vi "SetupDefault.vi"(8 "error in (no error)":errorcluster, 10 "Alias":string, 11 "SigGen_NIRF in":refnum<class "SigGen_NIRF.lvclass">) -> (0 "error out":errorcluster, 3 "SigGen_NIRF out":refnum<class "SigGen_NIRF.lvclass">)   [LabVIEW 2014, in "SigGen_NIRF.lvclass"]
uses:
  SigGen_NIRF.lvclass
  SigGen_NIRF.lvclass/SigGen_NIRF.ctl
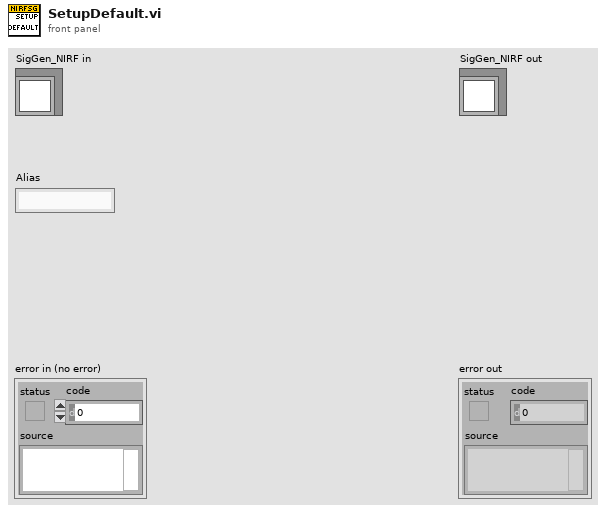
[diagram p1: front panel]
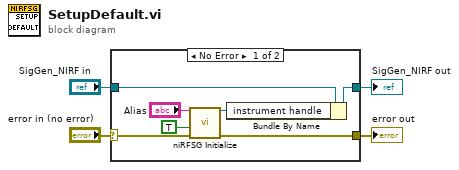
[diagram p0: block diagram]
diagram:
  n1 = case shown="No Error" "error in (no error)" {
    selector: "error in (no error)" -> [w5 w13]
    tunnel: "SigGen_NIRF in" -> [w10 w12]
    tunnel: [w9 w12] -> w3
    tunnel: [w7 w13] -> w2
    frame No Error {
      n2 = call "niRFSG Initialize.vi"("resource name"="Alias", "reset device"=TRUE, "error in"=w5) -> ("instrument handle"=w8:refnum<k15>, "error out"=w7:errorcluster)  [unwired: 11 in]
      n3 = Bundle By Name(cluster=w10, "instrument handle"=w8) -> (w9:refnum<class "SigGen_NIRF.lvclass">)
    }
    frame Error {
    }
  }
  "error out" <- w2
  "SigGen_NIRF out" <- w3
